vi "svx_Orbit Crosshair.vi"(4 "pen":T2={"Width"=2, "Style"=enum."Solid"}, 6 "crosshair color":u32(colorbox)=13055, 7 "crosshair size %":dbl=0.1, 10 "Plot Area:Size in":T1={"Width"=100, "Height"=100}, 11 "Picture in":picture) -> (2 "Plot Area:Size out":T1={"Width"=100, "Height"=100}, 3 "Picture out":picture)   [LabVIEW 2017, in "SVX Orbit.xctl"]
uses:
  <vilib>/addons/_XControls/Orbit Plot/SVX Orbit.xctl
  <vilib>/Utility/miscctls.llb/LVBoundsTypeDef.ctl
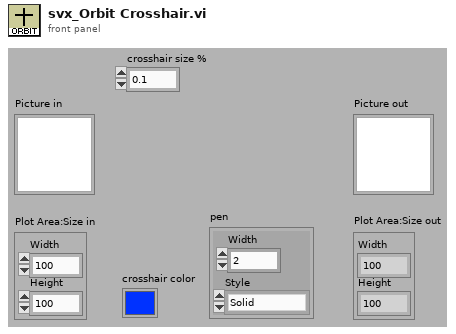
[diagram p1: front panel]
types:
  T1 = typedef "LVBoundsTypeDef.ctl" = cluster{"Width":u32, "Height":u32}
  T2 = cluster{"Width":u16, "Style":enum32{"Solid", "Dash", "Dot", "DashDot", "DashDotDot"}}
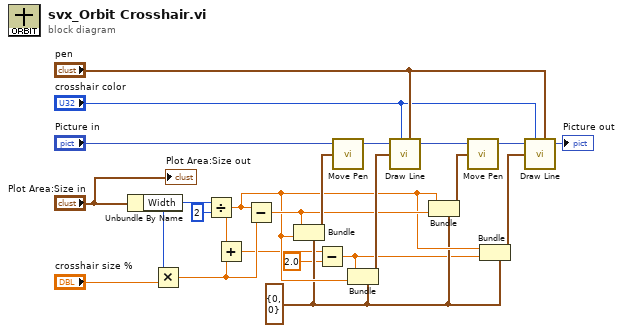
[diagram p0: block diagram]
diagram:
  w8 = cluster{"x":i16, "y":i16} {"x"=0, "y"=0} ("new position")
  n1 = Unbundle By Name("Plot Area:Size in") -> ("Width"=w20:u32)
  n2 = Multiply(x=w20, y="crosshair size %") -> (x*y=w17:dbl)
  n3 = Divide(x=w20, y=u32 2) -> (x/y=w10:dbl)
  n4 = Add(x=w10, y=w17) -> (x+y=w3:dbl)
  n5 = Subtract(x=w10, y=w17) -> (x-y=w12:dbl)
  n6 = Bundle(cluster=w8, "x"=w12, "y"=w10) -> (w18:cluster{"x":i16, "y":i16})
  n7 = Subtract(x=w3, y=2.0) -> (x-y=w1:dbl)
  n8 = call <vilib>:"Move Pen.vi"("new position"=w18, "picture"="Picture in") -> ("new picture"=w15:picture)  [unwired: 3 in]
  n9 = Bundle(cluster=w8, "x"=w1, "y"=w10) -> (w16:cluster{"x":i16, "y":i16})
  n10 = call <vilib>:"Draw Line.vi"("picture"=w15, "end point"=w16, "color(black)"="crosshair color", "pen"="pen") -> ("new picture"=w13:picture)  [unwired: 5 in]
  n11 = Bundle(cluster=w8, "x"=w10, "y"=w12) -> (w11:cluster{"x":i16, "y":i16})
  n12 = call <vilib>:"Move Pen.vi"("new position"=w11, "picture"=w13) -> ("new picture"=w14:picture)  [unwired: 3 in]
  n13 = Bundle(cluster=w8, "x"=w10, "y"=w1) -> (w9:cluster{"x":i16, "y":i16})
  n14 = call <vilib>:"Draw Line.vi"("picture"=w14, "end point"=w9, "color(black)"="crosshair color", "pen"="pen") -> ("new picture"=→"Picture out":picture)  [unwired: 5 in]
  "Plot Area:Size out" <- "Plot Area:Size in"
